vi "Motor X.vi"(10 "Magnitud Movimiento":i32, 11 "Direccion Movimiento":string) -> ()   [LabVIEW 2013, in "Proyecto 2 Touch.lvrbt"]
uses:
  Proyecto 2 Touch.lvrbt
  <vilib>/NXT/Block Support/NXT_OutputPort.ctl
  <vilib>/NXT/LegoClasses/BrickReference/BrickReference.lvclass
  <vilib>/NXT/Subs/LVHSConnector.ctl
  <vilib>/NXT/NXTIO Xnodes/NXTIONodeSubVIs/NXTMoveMotors.vi
  <vilib>/NXT/NXTIO Xnodes/NXTIOXNode/NXTIO.xnode
  <vilib>/NXT/NXTIO Xnodes/NXTIONodeSubVIs/LEGOResetMotors.vi
  <vilib>/NXT/NXTIO Xnodes/AddressXNode/NXTIOAddress.xnode
  <vilib>/NXT/NXTIO Xnodes/NXTIONodeSubVIs/LEGOStopAllMotors.vi
  <vilib>/NXT/Dual Mode Library/Waits/Wait_Rotation.vi
  <vilib>/NXT/Dual Mode Library/Waits/Wait_Num(msec).vi
  Global Var.vi
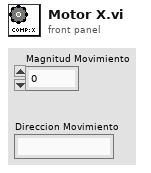
[diagram p1: front panel]
types:
  T1 = typedef "NXT_OutputPort.ctl" = u8
  T2 = typedef "LVHSConnector.ctl" = refnum<class "BrickReference.lvclass">
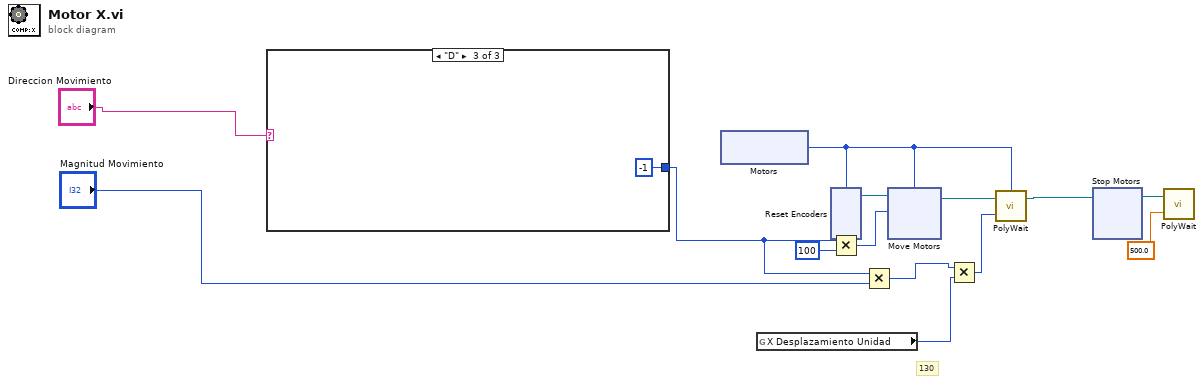
[diagram p0: block diagram]
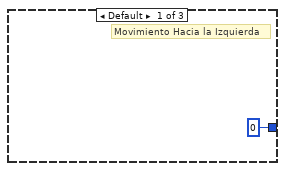
[diagram p2: hidden frame]
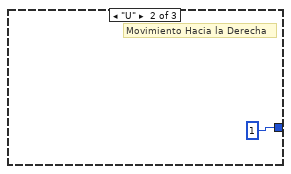
[diagram p3: hidden frame]
diagram:
  # "130"
  n1 = case shown="\"D\"" "Direccion Movimiento" {
    tunnel: [0 ("Magnitud Movimiento") 1 ("Magnitud Movimiento") -1 ("Magnitud Movimiento")] -> w3
    frame Default {
      # "Movimiento Hacia la Izquierda"
    }
    frame "U" {
      # "Movimiento Hacia la Derecha"
    }
    frame "D" {
    }
  }
  n2 = xnode "Motors"() -> ("Motor"=w7:T1)
  n3 = global read "Global Var.vi" "X Desplazamiento Unidad"() -> (w1:i32)
  n4 = xnode "Reset Encoders"("Motors"=w7) -> ("NXT/EV3"=w13:T2)  [unwired: 1 in]
  n5 = Multiply(x=w3, y=100) -> (x*y=w9:i32)
  n6 = Multiply(x=w3, y="Magnitud Movimiento") -> (x*y=w4:i32)
  n7 = xnode "Move Motors"("Power/Speed 1"=w9, "Motors"=w7, "NXT/EV3"=w13) -> ("NXT/EV3"=w10:T2)
  n8 = Multiply(x=w4, y=w1) -> (x*y=w8:i32)
  n9 = call-poly <vilib>:"PolyWait.vi"("Position Change (180)"=w8, "NXT/EV3"=w10, "Port (Port A)"=w7) -> ("NXT/EV3"=w6:T2)  [unwired: 1 in]
  n10 = xnode "Stop Motors"("NXT/EV3"=w6) -> ("NXT/EV3"=w12:T2)  [unwired: 1 in]
  n11 = call-poly <vilib>:"PolyWait.vi"("Time (100 msec)"=sgl 500.0 ("Time (1 sec)"), "NXT/EV3"=w12) -> ()  [unwired: 2 in, 1 out]
